vi "recupera_sesion_USB.vi"(7 "Espera acceso USB":u32, 11 "ftHandle_in":u32) -> (2 "ftHandle_out":u32, 3 "Valor Asic":u16 format="%x")   [LabVIEW 2019]
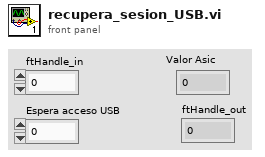
[diagram p1: front panel]
types:
  T1 = cluster{"Device Index":u32, "FT_FLAGS_OPENED":bool, "FT_FLAGS_HISPEED":bool, "Type":u32, "VID":u32, "PID":u32, "LocID":i32, "Serial Number":string, "Description":string, "FT_Handle":u32}
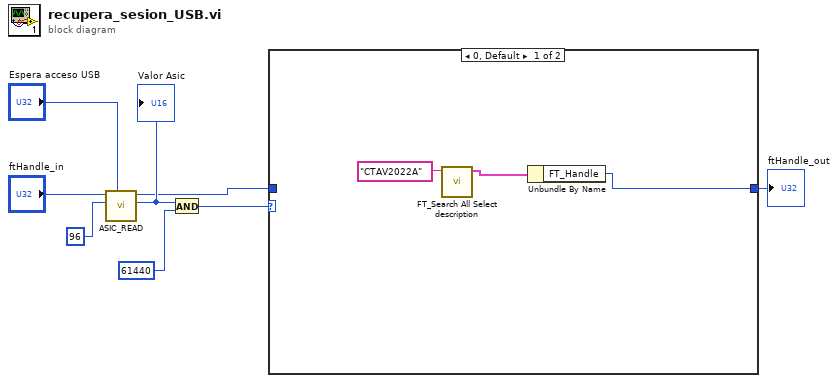
[diagram p0: block diagram]
diagram:
  n1 = call "ASIC_READ.vi"("Espera acceso USB"="Espera acceso USB", "Direccion Registro Asic"=u8 96, "ftHandle_in"="ftHandle_in") -> ("Valor Asic"=w5:u16, "ftHandle_out"=w2:u32)  [unwired: 6 in, 1 out]
  "Valor Asic" <- w5
  n2 = And(x=w5, y=u16 61440) -> (x .and. y?=w3:u16)
  n3 = case shown="0, Default" w3 {
    tunnel: w2 -> [_ w12]
    tunnel: [w10 w12] -> w1
    frame 0, Default {
      n4 = call "FT_Search All Select description.vi"("CTA Test#"="CTAV2022A") -> ("Select Ft"=w11:T1)  [unwired: 8 in, 2 out]
      n5 = Unbundle By Name(w11) -> ("FT_Handle"=w10:u32)
    }
    frame 16384, 20480, 24576 {
    }
  }
  "ftHandle_out" <- w1
